vi "Set Sequence.vi"(5 "timeout ms (-1)":i32=-1, 6 "Station":T1(ring), 8 "error in (no error)":errorcluster, 11 "Sequence":string) -> (0 "error out":errorcluster)   [LabVIEW 2019, in "Test Bench Tools.lvlib"]
uses:
  Test Bench Tools.lvlib
  TB Global 1.vi
  <resource>/objmgr/ni.dex.rc
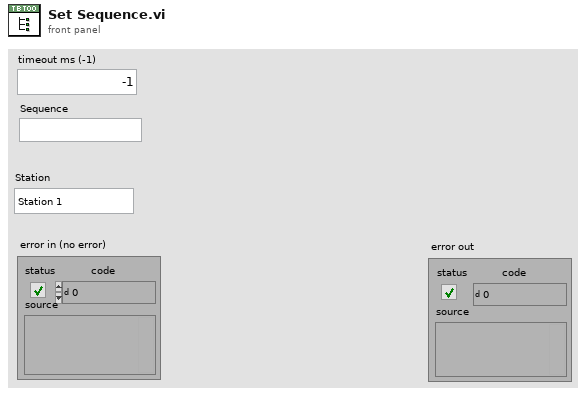
[diagram p1: front panel]
types:
  T1 = enum16{"Station 1", "Station 2", "Station 3", "Station 4"}
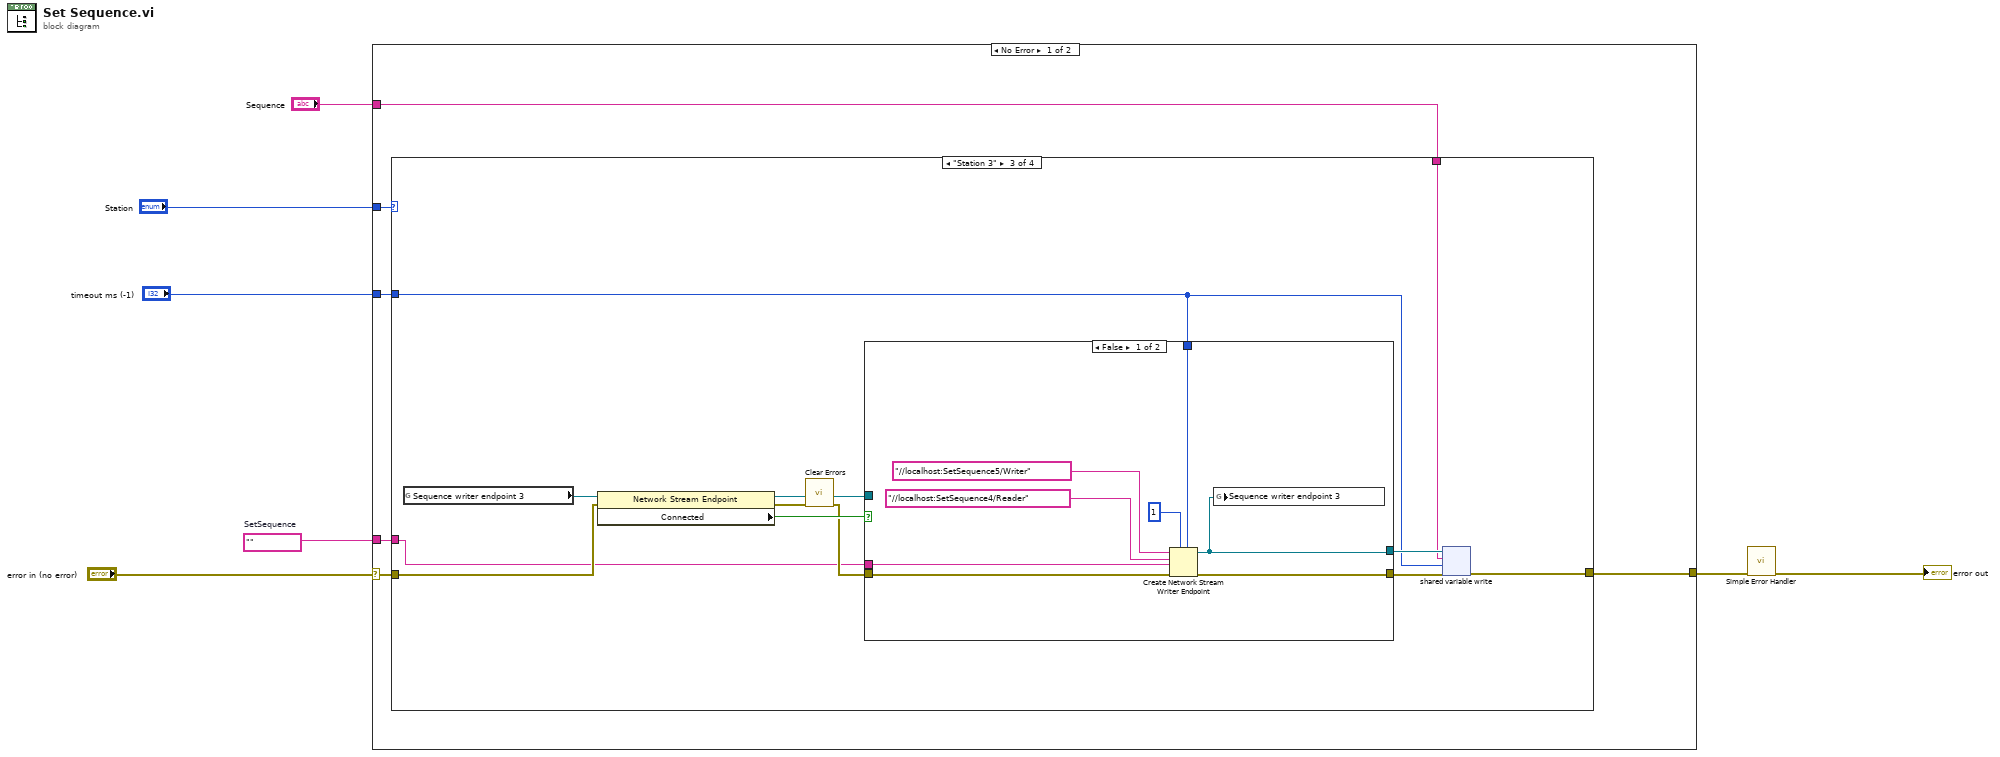
[diagram p0: block diagram]
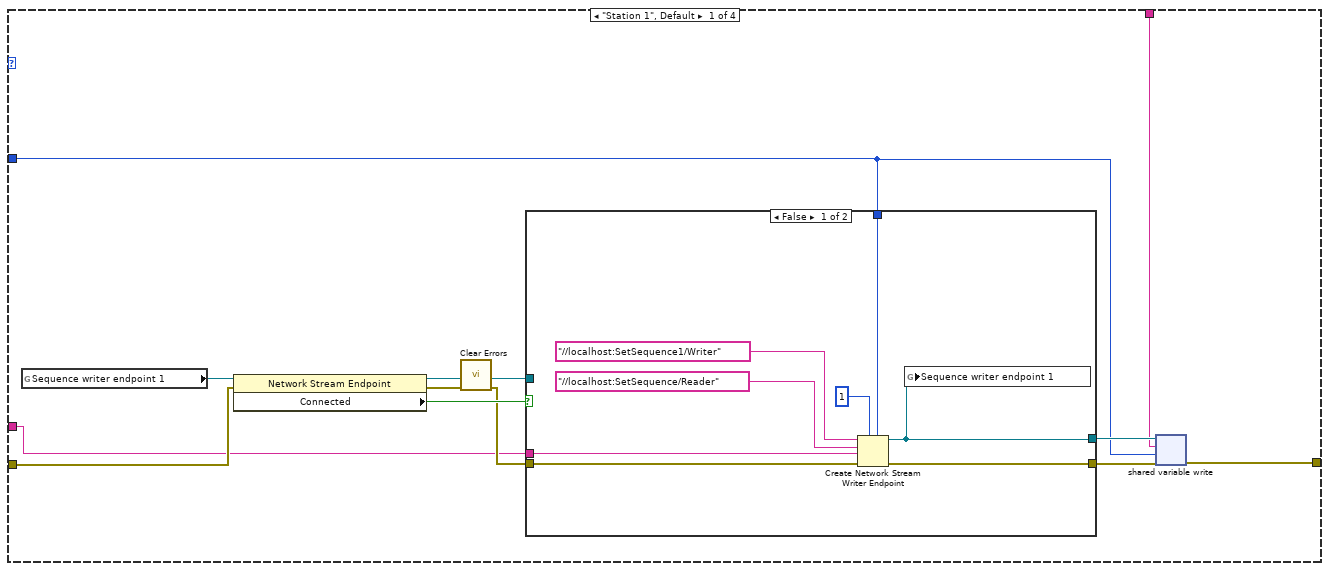
[diagram p2: hidden frame]
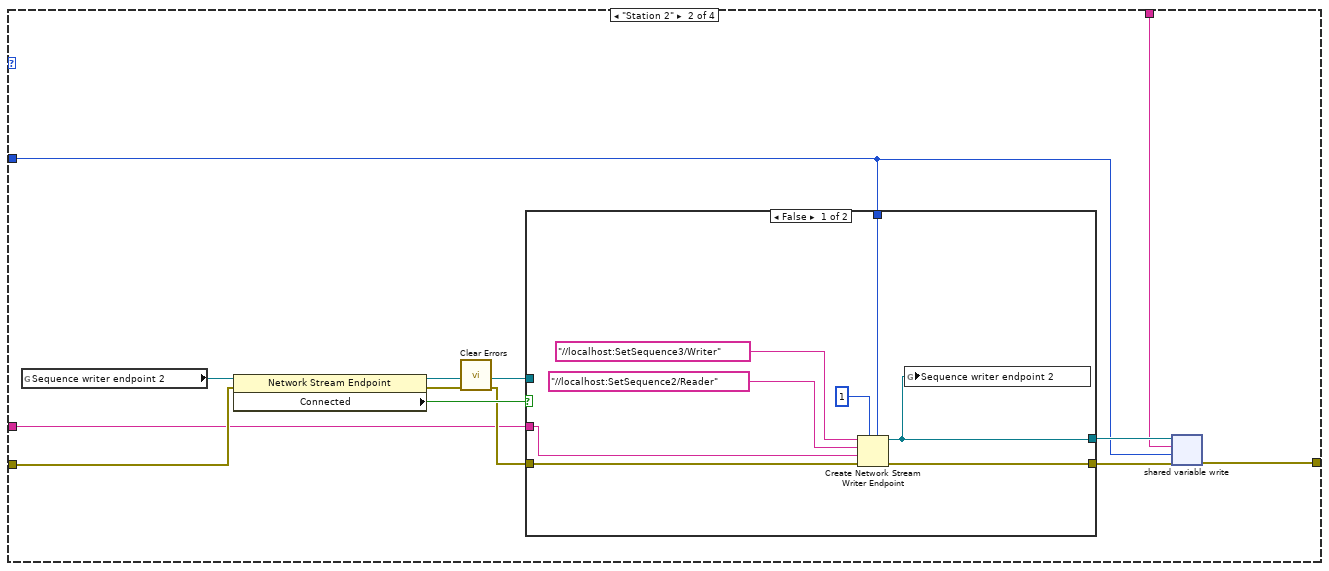
[diagram p4: hidden frame]
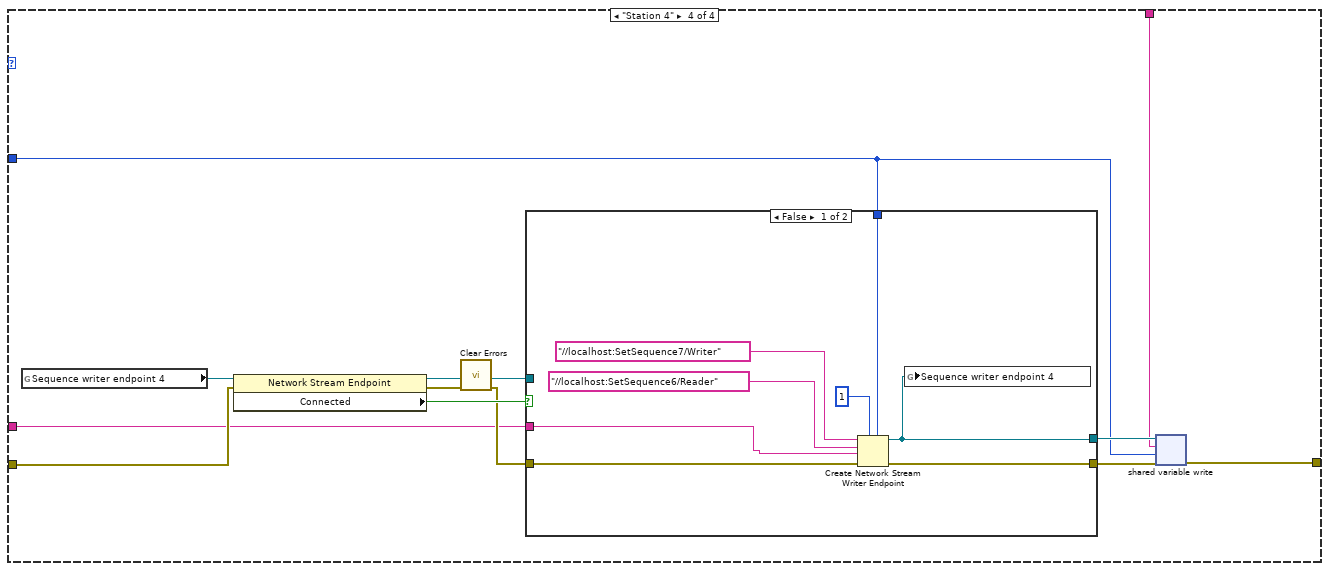
[diagram p7: hidden frame]
diagram:
  w2 = ""  # SetSequence
  n1 = case shown="No Error" "error in (no error)" {
    selector: "error in (no error)" -> [w12 w102]
    tunnel: "timeout ms (-1)" -> [w11 _]
    tunnel: "Sequence" -> [w10 _]
    tunnel: [w13 w102] -> w6
    tunnel: "Station" -> [w9 _]
    tunnel: w2 -> [w8 _]
    frame No Error {
      n2 = case shown="\"Station 3\"" w9 {
        tunnel: [w19 w41 w63 w85] -> w13
        tunnel: w12 -> [w18 w40 w62 w84]
        tunnel: w11 -> [w16 w38 w60 w82]
        tunnel: w10 -> [w15 w37 w59 w81]
        tunnel: w8 -> [w14 w36 w58 w80]
        frame "Station 1", Default {
          n3 = global read "TB Global 1.vi" "Sequence writer endpoint 1"() -> (w23:refnum<k21>)
          n4 = property class="Network Stream Endpoint"(reference=w23, error in=w18) -> (reference out=w20:refnum<k21>, error out=w22:errorcluster, "Connected"=w21:bool)
          n5 = call <vilib>:"Clear Errors.vi"("error in (no error)"=w22) -> ("error out"=w17:errorcluster)  [unwired: 5 in, 1 out]
          n6 = case shown="False" w21 {
            tunnel: [w26 w35] -> w25
            tunnel: [w28 w34] -> w24
            tunnel: w17 -> [w30 w34]
            tunnel: w20 -> [_ w35]
            tunnel: w16 -> [w29 _]
            tunnel: w14 -> [w27 _]
            frame False {
              n7 = Create Network Stream Writer Endpoint(5:w29, 7:1 ("writer buffer size"), 8:w30, 9:w27, 10:"//localhost:SetSequence/Reader" ("reader name"), 11:"//localhost:SetSequence1/Writer" ("reader name")) -> (0:w28:errorcluster, 3:w26:refnum<k21>)  [unwired: 1 in]
              n8 = global write "TB Global 1.vi" "Sequence writer endpoint 1"(w26) -> ()
            }
            frame True {
            }
          }
          n9 = shared-variable-write(w25, w24, w15, w16) -> (w19:errorcluster)  [unwired: 2 out]
        }
        frame "Station 2" {
          n10 = global read "TB Global 1.vi" "Sequence writer endpoint 2"() -> (w45:refnum<k21>)
          n11 = property class="Network Stream Endpoint"(reference=w45, error in=w40) -> (reference out=w42:refnum<k21>, error out=w44:errorcluster, "Connected"=w43:bool)
          n12 = call <vilib>:"Clear Errors.vi"("error in (no error)"=w44) -> ("error out"=w39:errorcluster)  [unwired: 5 in, 1 out]
          n13 = case shown="False" w43 {
            tunnel: [w49 w57] -> w47
            tunnel: [w50 w56] -> w46
            tunnel: w39 -> [w52 w56]
            tunnel: w42 -> [_ w57]
            tunnel: w38 -> [w51 _]
            tunnel: w36 -> [w48 _]
            frame False {
              n14 = Create Network Stream Writer Endpoint(5:w51, 7:1 ("writer buffer size"), 8:w52, 9:w48, 10:"//localhost:SetSequence2/Reader" ("reader name"), 11:"//localhost:SetSequence3/Writer" ("reader name")) -> (0:w50:errorcluster, 3:w49:refnum<k21>)  [unwired: 1 in]
              n15 = global write "TB Global 1.vi" "Sequence writer endpoint 2"(w49) -> ()
            }
            frame True {
            }
          }
          n16 = shared-variable-write(w47, w46, w37, w38) -> (w41:errorcluster)  [unwired: 2 out]
        }
        frame "Station 3" {
          n17 = global read "TB Global 1.vi" "Sequence writer endpoint 3"() -> (w67:refnum<k21>)
          n18 = property class="Network Stream Endpoint"(reference=w67, error in=w62) -> (reference out=w64:refnum<k21>, error out=w66:errorcluster, "Connected"=w65:bool)
          n19 = call <vilib>:"Clear Errors.vi"("error in (no error)"=w66) -> ("error out"=w61:errorcluster)  [unwired: 5 in, 1 out]
          n20 = case shown="False" w65 {
            tunnel: [w71 w79] -> w69
            tunnel: [w72 w78] -> w68
            tunnel: w61 -> [w74 w78]
            tunnel: w64 -> [_ w79]
            tunnel: w60 -> [w73 _]
            tunnel: w58 -> [w70 _]
            frame False {
              n21 = Create Network Stream Writer Endpoint(5:w73, 7:1 ("writer buffer size"), 8:w74, 9:w70, 10:"//localhost:SetSequence4/Reader" ("reader name"), 11:"//localhost:SetSequence5/Writer" ("reader name")) -> (0:w72:errorcluster, 3:w71:refnum<k21>)  [unwired: 1 in]
              n22 = global write "TB Global 1.vi" "Sequence writer endpoint 3"(w71) -> ()
            }
            frame True {
            }
          }
          n23 = shared-variable-write(w69, w68, w59, w60) -> (w63:errorcluster)  [unwired: 2 out]
        }
        frame "Station 4" {
          n24 = global read "TB Global 1.vi" "Sequence writer endpoint 4"() -> (w89:refnum<k21>)
          n25 = property class="Network Stream Endpoint"(reference=w89, error in=w84) -> (reference out=w86:refnum<k21>, error out=w88:errorcluster, "Connected"=w87:bool)
          n26 = call <vilib>:"Clear Errors.vi"("error in (no error)"=w88) -> ("error out"=w83:errorcluster)  [unwired: 5 in, 1 out]
          n27 = case shown="False" w87 {
            tunnel: [w93 w101] -> w91
            tunnel: [w94 w100] -> w90
            tunnel: w83 -> [w96 w100]
            tunnel: w86 -> [_ w101]
            tunnel: w82 -> [w95 _]
            tunnel: w80 -> [w92 _]
            frame False {
              n28 = Create Network Stream Writer Endpoint(5:w95, 7:1 ("writer buffer size"), 8:w96, 9:w92, 10:"//localhost:SetSequence6/Reader" ("reader name"), 11:"//localhost:SetSequence7/Writer" ("reader name")) -> (0:w94:errorcluster, 3:w93:refnum<k21>)  [unwired: 1 in]
              n29 = global write "TB Global 1.vi" "Sequence writer endpoint 4"(w93) -> ()
            }
            frame True {
            }
          }
          n30 = shared-variable-write(w91, w90, w81, w82) -> (w85:errorcluster)  [unwired: 2 out]
        }
      }
    }
    frame Error {
    }
  }
  n31 = call <vilib>:"Simple Error Handler.vi"("error in (no error)"=w6) -> ("error out"=→"error out":errorcluster)  [unwired: 4 in, 4 out]
